vi "RemoteControl.TestLauncher.Client3.vi"() -> ()   [LabVIEW 2016, in "RemoteControl.lvclass"]
uses:
  RemoteControl.lvclass
  <vilib>/JKI/JKI SMO/SMO/Typedefs/SMOState --Enum.ctl
  Typedefs/Message--Cluster.ctl
  C:/Program Files (x86)/National Instruments/LabVIEW 2016/vi.lib/JKI/JKI SMO/SMO/SMO.lvclass
  RemoteControl.STM/RemoteControl.STM.lvclass
  C:/user/patrick/hg/levylab_inst/lvsrc/SMOs/RemoteControl/RemoteControl.lvclass
  Typedefs/PrivateEvents--RemoteControl.SendMessageToProcess.ctl
  <vilib>/JKI/JKI SMO/SMO/SMO.lvclass
panel:
  out "x-y":i32
  in  "timeout":i32=50
  out "received":i32
  out "sent":i32
  in  "Send?":bool
  out "Message Sent":T1
  out "Message Received":T1
  in  "T = STM":bool
  in  "Message to Send":T1
  in  "Port":u32=6341
  in  "Address":string
  out "SMO State":T2
  out "error out":errorcluster
  in  "Stop":bool
  # "SM SMO Test Launcher: Client 3"
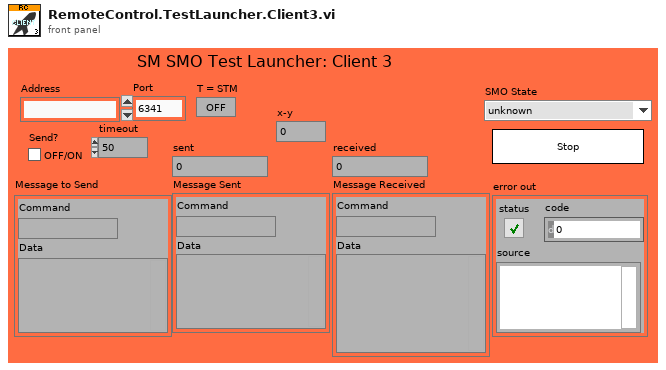
[diagram p1: front panel]
types:
  T1 = typedef "RemoteControl.lvclass/Message--Cluster.ctl" = cluster{"Command":string, "Data":variant}
  T2 = typedef "SMO.lvclass/SMOState --Enum.ctl" = enum16{"unknown", "Created", "Started", "Stopped"}
  T3 = typedef "SMO.lvclass/Public Events.ctl" = cluster{"Error":refnum<user-event>, "State":refnum<user-event>, "Reserve State":refnum<user-event>}
  T4 = typedef "RemoteControl.lvclass/PublicEvents--Cluster.ctl" = cluster{"SendMessageFromProcess":refnum<user-event>}
  T5 = typedef "RemoteControl.lvclass/PrivateEvents--RemoteControl.SendMessageToProcess.ctl" = cluster{"Message":T1, "Message ID":u32}
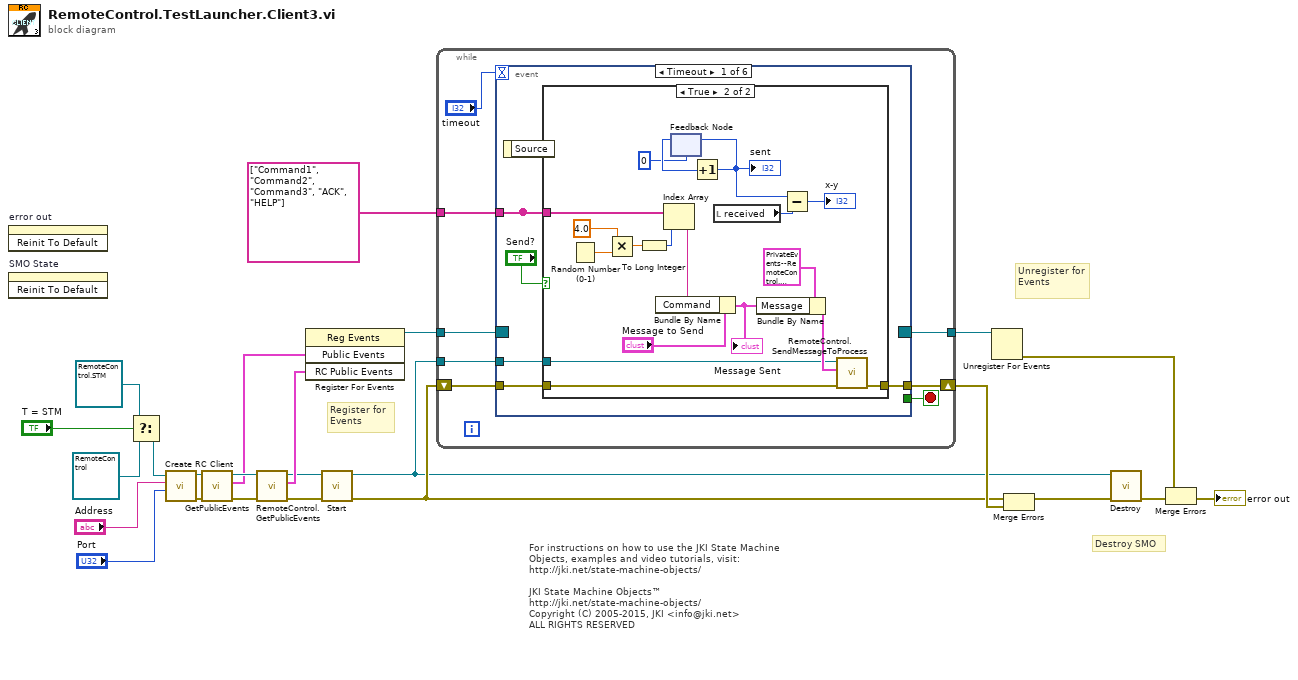
[diagram p0: block diagram]
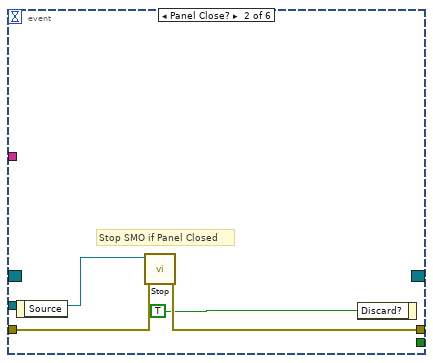
[diagram p3: hidden frame]
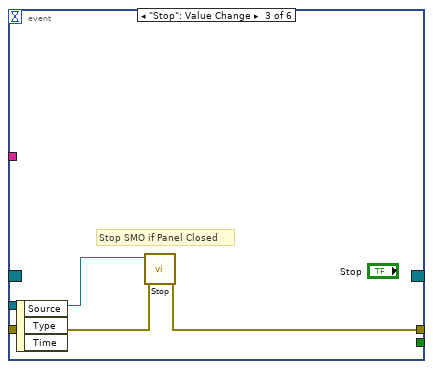
[diagram p4: hidden frame]
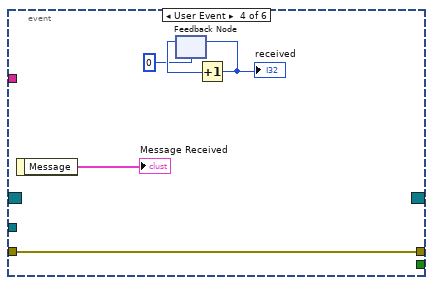
[diagram p5: hidden frame]
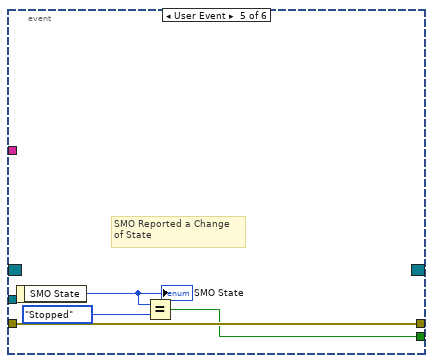
[diagram p6: hidden frame]
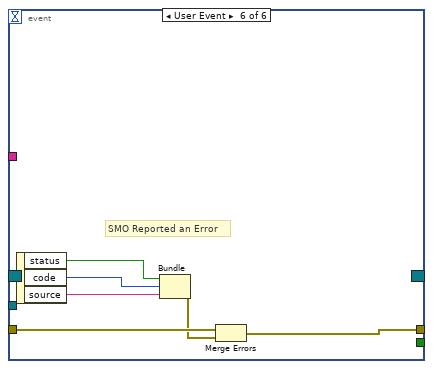
[diagram p7: hidden frame]
diagram:
  # "For instructions on how to use the JKI State Machine Objects, examples and video tutorials, visit:\nhttp://jki.net/state-machine-objects/\n\nJKI State Machine Objects™\nhttp://jki.net/state-machine-objects/\nCopyright (C) 2005-2015, JKI <info@jki.net>\nALL RIGHTS RESERVED"
  # "Destroy SMO"
  # "Unregister for Events"
  # "Register for Events"
  n1 = invoke on="error out" class="Clust (strict)" method="Reinit To Default"() -> ()  [unwired: 3 in, 3 out]
  n2 = invoke on="SMO State" class="Enum (strict)" method="Reinit To Default"() -> ()  [unwired: 3 in, 3 out]
  n3 = Select(t=refnum<class "RemoteControl.STM.lvclass"> refnum ("RemoteControl.STM.lvclass"), s="T = STM", f=refnum<class "RemoteControl.lvclass"> refnum ("SMO.Template.lvclass")) -> (s? t:f=w13:refnum<class "RemoteControl.lvclass">)
  n4 = call-dynamic "Create RC Client.vi"("Port"="Port", "Address"="Address", "RemoteControl in"=w13) -> ("error out"=w12:errorcluster, "RemoteControl out"=w11:refnum<class "RemoteControl.lvclass">)  [unwired: 7 in]
  n5 = call <vilib>:"GetPublicEvents.vi"("error in (no error)"=w12, "SMO"=w11) -> ("error out"=w9:errorcluster, "Public Events"=w8:T3, "SMO out"=w10:refnum<class "RemoteControl.lvclass">)  [unwired: 7 in]
  n6 = call "RemoteControl.GetPublicEvents.vi"("error in (no error)"=w9, "RemoteControl"=w10) -> ("error out"=w4:errorcluster, "RC Public Events"=w7:T4, "RemoteControl out"=w5:refnum<class "RemoteControl.lvclass">)  [unwired: 7 in]
  n7 = register-events(w8, w7) -> (reference out=w6:refnum<event-registration>)  [unwired: 2 in, 1 out]
  n8 = call <vilib>:"Start.vi"("error in (no error)"=w4, "SMO"=w5) -> ("error out"=w3:errorcluster, "SMO out"=w2:refnum<class "RemoteControl.lvclass">)  [unwired: 8 in]
  n9 = while {
    shift-right: [w31] -> w23
    shift-left: w3 -> [w30]
    tunnel: w6 -> [w29]
    tunnel: [w28] -> w24
    tunnel: w2 -> [w27]
    tunnel: string[] ["Command1", "Command2", "Command3", "ACK", "HELP"] ("Commands") -> [w25]
    stop <- w32 stop-if-true
    n10 = event shown="[0] Timeout" {
      selector: w29 -> [_ _ _ _ _ _]
      dyn-events: [_ _ _ _ _ _] -> w28
      timeout: "timeout" -> [_ _ _ _ _ _]
      tunnel: [_ _ _ _ w69 _] -> w32
      tunnel: w27 -> [w36 w60 w63 _ _ _]
      tunnel: [w35 w59 w62 w68 w72 w76] -> w31
      tunnel: w30 -> [w37 w58 w61 w68 w72 w74]
      tunnel: [w34 _ _ _ _ _] -> _
      tunnel: w25 -> [w34 _ _ _ _ _]
      event Timeout {
        n11 = event-data() -> ()  [unwired: 1 in, 1 out]
        n12 = case shown="True" "Send?" {
          tunnel: w37 -> [w38 w54]
          tunnel: w36 -> [_ w53]
          tunnel: [w38 w52] -> w35
          tunnel: w34 -> [_ w42]
          frame False {
          }
          frame True {
            n13 = Random Number (0-1)() -> (number: 0 to 1=w51:dbl)
            n14 = Multiply(x=4.0, y=w51) -> (x*y=w50:dbl)
            n15 = To Long Integer(number=w50) -> (32bit integer=w49:i32)
            n16 = Index Array(array=w42, index=w49) -> (element=w43:string)
            n17 = Bundle By Name(cluster="Message to Send", "Command"=w43) -> (w48:T1)
            "Message Sent" <- w48
            n18 = feedback #1(0) -> (w45:i32)
            n19 = Increment(x=w45) -> (x+1=w39:i32)
            "sent" <- w39
            n20 = feedback-in #1(w39) -> ()
            n21 = local read "received"() -> (w41:i32)
            n22 = Bundle By Name(cluster=T5 {"Message"={"Command"="", "Data"=variant(bool FALSE)}, "Message ID"=0} ("SendMessgaeToProcess"), "Message"=w48) -> (w55:T5)
            n23 = Subtract(x=w39, y=w41) -> (x-y=→"x-y":i32)
            n24 = call "RemoteControl.SendMessageToProcess.vi"("error in (no error)"=w54, "SendMessgaeToProcess"=w55, "RemoteControl"=w53) -> ("error out"=w52:errorcluster)  [unwired: 7 in, 1 out]
          }
        }
      }
      event Panel Close? {
        # "Stop SMO if Panel Closed"
        n25 = event-data() -> ()  [unwired: 1 in, 1 out]
        n26 = call <vilib>:"Stop.vi"("error in (no error)"=w58, "SMO"=w60) -> ("error out"=w59:errorcluster)  [unwired: 8 in, 1 out]
        n27 = event-data("Discard?"=TRUE ("OK")) -> ()  [unwired: 1 in, 1 out]
      }
      event "Stop": Value Change {
        # "Stop SMO if Panel Closed"
        n28 = event-data() -> ()  [unwired: 1 in, 3 out]
        n29 = call <vilib>:"Stop.vi"("error in (no error)"=w61, "SMO"=w63) -> ("error out"=w62:errorcluster)  [unwired: 8 in, 1 out]
      }
      event User Event {
        n30 = event-data() -> ("Message"=→"Message Received":T1)  [unwired: 1 in]
        n31 = feedback #2(0) -> (w65:i32)
        n32 = Increment(x=w65) -> (x+1=w66:i32)
        "received" <- w66
        n33 = feedback-in #2(w66) -> ()
      }
      event User Event {
        # "SMO Reported a Change\nof State"
        n34 = event-data() -> ("SMO State"=w71:T2)  [unwired: 1 in]
        "SMO State" <- w71
        n35 = Equal?(x=w71, y=SMOState_--Enum."Stopped") -> (x = y?=w69:bool)
      }
      event User Event {
        # "SMO Reported an Error"
        n36 = event-data() -> ("status"=w75:bool, "code"=w78:i32, "source"=w77:string)  [unwired: 1 in]
        n37 = Bundle("status"=w75, "code"=w78, "source"=w77) -> (w73:errorcluster)  [unwired: 1 in]
        n38 = Merge Errors(w74, w73) -> (w76:errorcluster)
      }
    }
  }
  n39 = Unregister For Events(event registration refnum=w24) -> (error out=w22:errorcluster)  [unwired: 1 in]
  n40 = Merge Errors(w3, w23) -> (w19:errorcluster)
  n41 = call <vilib>:"Destroy.vi"("error in (no error)"=w19, "SMO"=w2) -> ("error out"=w20:errorcluster)  [unwired: 9 in]
  n42 = Merge Errors(w22, w20) -> (→"error out":errorcluster)
